vi "tipshapingstr (SubVI).vi"(11 "Array":string[](array[string])) -> (5 "String":string)   [LabVIEW 2014]
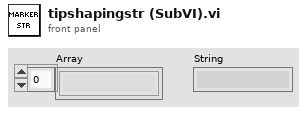
[diagram p1: front panel]
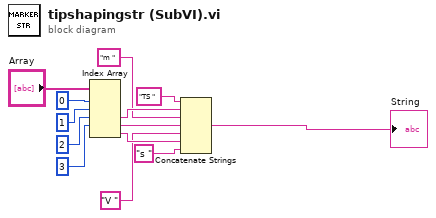
[diagram p0: block diagram]
diagram:
  n1 = Index Array(array="Array", index #1=0 ("index"), index #2=1 ("index"), index #3=2 ("index"), index #4=3 ("index")) -> (element #3=w12:string, element #4=w5:string, element #5=w4:string)  [unwired: 1 in, 2 out]
  n2 = Concatenate Strings("TS " ("string"), w12, "m " ("string"), w5, "V " ("string"), w4, "s " ("string")) -> (→"String":string)
